vi "HalfDrive.vi"(7 "Scaler":dbl=1.0 min=0.0 max=1.0 step=0.05 format="%#_13g", 9 "RightDrive in":dbl, 10 "LeftDrive in":dbl, 11 "HalfDrive":bool) -> (1 "RightDrive out":dbl, 2 "LeftDrive out":dbl)   [LabVIEW 2015]
doc: "Cuts the motor values in half if HalfDrive is true."
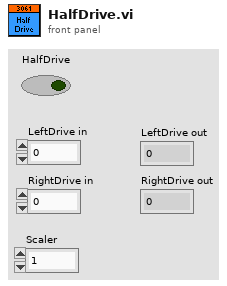
[diagram p1: front panel]
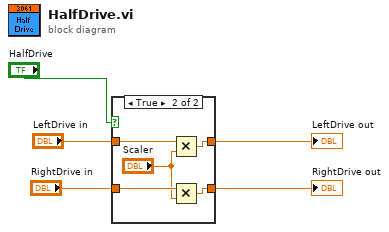
[diagram p0: block diagram]
diagram:
  n1 = case shown="True" "HalfDrive" {
    tunnel: "LeftDrive in" -> [w7 w12]
    tunnel: "RightDrive in" -> [w6 w11]
    tunnel: [w7 w9] -> w3
    tunnel: [w6 w8] -> w2
    frame False {
    }
    frame True {
      n2 = Multiply(x=w12, y="Scaler") -> (x*y=w9:dbl)
      n3 = Multiply(x=w11, y="Scaler") -> (x*y=w8:dbl)
    }
  }
  "LeftDrive out" <- w3
  "RightDrive out" <- w2
